vi "LJM_CloseAll.vi"(8 "error in":errorcluster) -> (0 "error out":errorcluster)   [LabVIEW 2024]
uses:
  labjackm.dll
panel:
  # "Calls CloseAll even if error in is true."
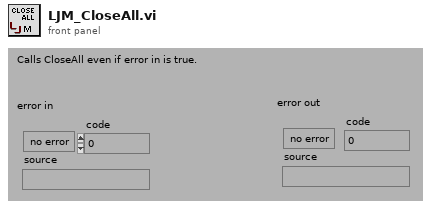
[diagram p1: front panel]
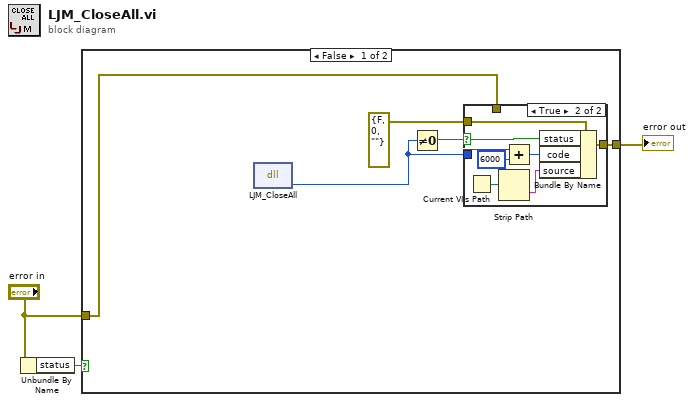
[diagram p0: block diagram]
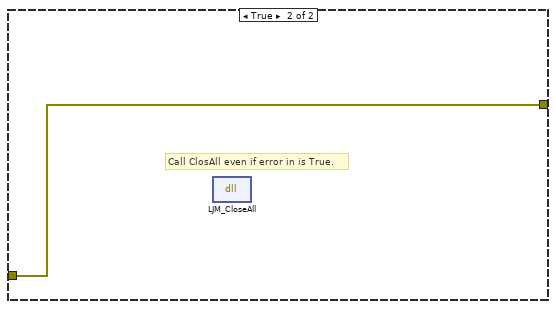
[diagram p3: hidden frame]
diagram:
  n1 = Unbundle By Name("error in") -> ("status"=w2:bool)
  n2 = case shown="False" w2 {
    tunnel: [w5 w18] -> w3
    tunnel: "error in" -> [w4 w18]
    frame False {
      n3 = dll-call lib="labjackm.dll" fn="LJM_CloseAll"() -> (w6:i32)  [unwired: 3 in, 2 out]
      n4 = Not Equal To 0?(x=w6) -> (x != 0?=w7:bool)
      n5 = case shown="True" w7 {
        selector: w7 -> [_ w16]
        tunnel: [w9 w17] -> w5
        tunnel: errorcluster {"status"=FALSE, "code"=0, "source"=""} ("error IO") -> [_ w15]
        tunnel: w6 -> [_ w11]
        tunnel: w4 -> [w9 _]
        frame False {
        }
        frame True {
          n6 = Current VI's Path() -> (path=w13:path)
          n7 = Strip Path(path=w13) -> (name=w14:string)  [unwired: 1 out]
          n8 = Add(x=w11, y=6000) -> (x+y=w12:i32)
          n9 = Bundle By Name(cluster=w15, "status"=w16, "code"=w12, "source"=w14) -> (w17:errorcluster)
        }
      }
    }
    frame True {
      # "Call ClosAll even if error in is True."
      n10 = dll-call lib="labjackm.dll" fn="LJM_CloseAll"() -> ()  [unwired: 4 in, 2 out]
    }
  }
  "error out" <- w3
